vi "avg joystick and frame trig lick3.vi"(10 "stop in":refnum<vi>, 11 "Joystick File":path=path "C:/Users/Mackenzie Amoroso/Desktop/junk") -> ()   [LabVIEW 2017]
uses:
  <vilib>/DAQmx/read.llb/DAQmx Read (Analog 2D DBL NChan NSamp).vi
  PushTask Globals.vi
  <vilib>/DAQmx/miscellaneous.llb/DAQmx Fill In Error Info.vi
  <resource>/objmgr/daqmx.rc
panel:
  out "frame count 2":u32
  in  "stop 2":bool
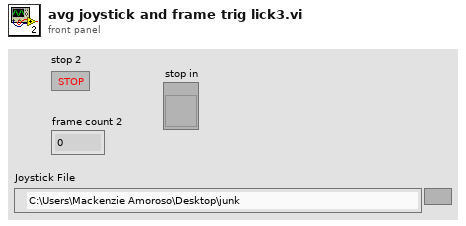
[diagram p1: front panel]
types:
  T1 = enum16{"open", "replace", "create", "open or create", "replace or create", "replace or create with confirmation"}
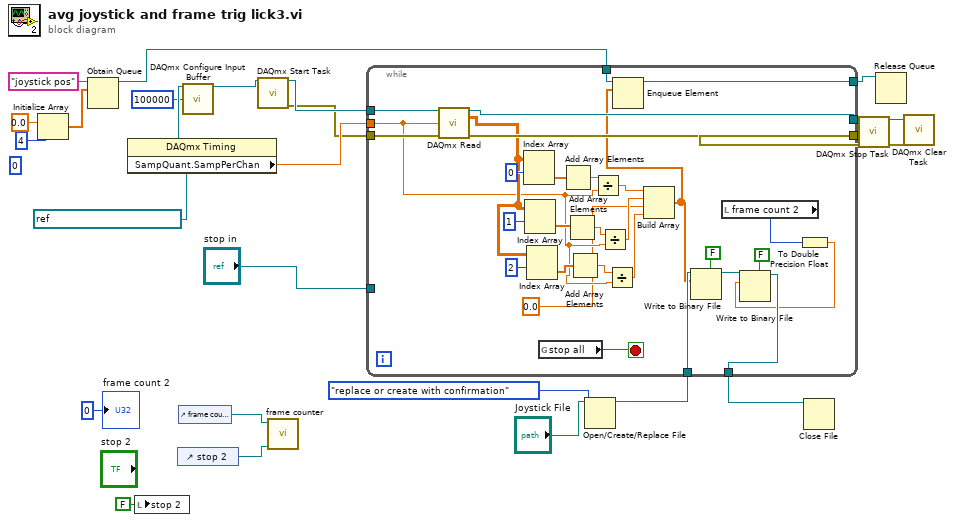
[diagram p0: block diagram]
diagram:
  (unwired) 0 ("dimension size")
  n1 = Initialize Array(0.0 ("element"), 4 ("dimension size")) -> (w15:dbl[])
  n2 = Obtain Queue(name (unnamed)="joystick pos", element data type=w15) -> (queue out=w14:refnum<queue>)  [unwired: 3 in, 2 out]
  n3 = property class="DAQmx Timing"(reference=refnum<k21> "joysticklickframe_push" ("task/channels in")) -> (reference out=w3:refnum<k21>, "SampQuant.SampPerChan"=w22:dbl)  [unwired: 1 in, 1 out]
  n4 = local write "stop 2"(FALSE ("stop")) -> ()
  n5 = control-ref of="stop 2"() -> (w6:refnum<vi>)
  n6 = control-ref of="frame count 2"() -> (w7:refnum<vi>)
  n7 = call <vilib>:"DAQmx Configure Input Buffer.vi"("task/channels in"=w3, "buffer size (in samples per channel)"=u32 100000) -> ("task out"=w2:refnum<k21>)  [unwired: 12 in, 1 out]
  n8 = call <vilib>:"DAQmx Start Task.vi"("task/channels in"=w2) -> ("task out"=w24:refnum<k21>, "error out"=w21:errorcluster)  [unwired: 13 in]
  n9 = call "frame counter.vi"("stop ref"=w6, "frame count ref"=w7) -> ()  [unwired: 10 in]
  n10 = Open/Create/Replace File(file path (use dialog)="Joystick File", operation (0:open)=T1."replace or create with confirmation") -> (refnum out=w10:refnum<file>)  [unwired: 4 in, 2 out]
  n11 = while {
    tunnel: w24 -> [w56]
    tunnel: w22 -> [w35]
    tunnel: w21 -> [w55]
    tunnel: [w54] -> w20
    tunnel: [w53] -> w19
    tunnel: w14 -> [w45]
    tunnel: [w43] -> w13
    tunnel: w10 -> [w42]
    tunnel: [w32] -> w9
    tunnel: "stop in" -> [_]
    stop <- w29 stop-if-true
    n12 = call-poly <vilib>:"DAQmx Read.vi"("task/channels in"=w56, "number of samples per channel"=w35, "error in"=w55) -> ("task out"=w54:refnum<k21>, "data"=w36:dbl[][], "error out"=w53:errorcluster)  [unwired: 10 in]
    n13 = Index Array(array=w36, index (row)=0) -> (element=w50:dbl[])  [unwired: 1 in]
    n14 = Index Array(array=w36, index (row)=1) -> (element=w49:dbl[])  [unwired: 1 in]
    n15 = Index Array(array=w36, index (row)=2) -> (element=w39:dbl[])  [unwired: 1 in]
    n16 = global read "PushTask Globals.vi" "stop all"() -> (w29:bool)
    n17 = Add Array Elements(numeric array=w50) -> (sum=w48:dbl)
    n18 = Add Array Elements(numeric array=w49) -> (sum=w47:dbl)
    n19 = Add Array Elements(numeric array=w39) -> (sum=w38:dbl)
    n20 = Divide(x=w48, y=w35) -> (x/y=w46:dbl)
    n21 = Divide(x=w47, y=w35) -> (x/y=w44:dbl)
    n22 = Divide(x=w38, y=w35) -> (x/y=w28:dbl)
    n23 = Build Array(w46, w44, 0.0 ("element"), w28) -> (w37:dbl[])
    n24 = Enqueue Element(queue=w45, element=w37) -> (queue out=w43:refnum<queue>)  [unwired: 2 in, 2 out]
    n25 = Write to Binary File(file (use dialog)=w42, data=w37, 5:FALSE ("prepend array or string size? (T)")) -> (refnum out=w33:refnum<file>)  [unwired: 3 in, 2 out]
    n26 = local read "frame count 2"() -> (w31:u32)
    n27 = To Double Precision Float(number=w31) -> (double precision float=w30:dbl)
    n28 = Write to Binary File(file (use dialog)=w33, data=w30, 5:FALSE ("prepend array or string size? (T)")) -> (refnum out=w32:refnum<file>)  [unwired: 3 in, 2 out]
  }
  n29 = Close File(refnum=w9) -> ()  [unwired: 1 in, 2 out]
  n30 = call <vilib>:"DAQmx Stop Task.vi"("task/channels in"=w20, "error in"=w19) -> ("task out"=w26:refnum<k21>, "error out"=w25:errorcluster)  [unwired: 12 in]
  n31 = Release Queue(queue=w13) -> ()  [unwired: 2 in, 3 out]
  n32 = call <vilib>:"DAQmx Clear Task.vi"("task in"=w26, "error in"=w25) -> ()  [unwired: 13 in, 1 out]
  "frame count 2" <- u32 0 ("frame count")
